vi "Read Digital Input and Output Module.vi"   [LabVIEW 2017, in "Scan Engine Scripting.lvlib"]
doc: "Returns the channel settings of a digital input and output module that can be edited and then used to create a new module instance to set into a slot."
uses:
  Scan Engine Scripting.lvlib
  NI 9375/NI 9375.lvclass
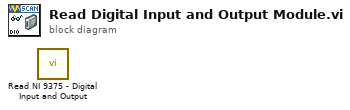
[diagram p0: block diagram]
diagram:
  n1 = call "Read NI 9375 - Digital Input and Output.vi"() -> ()  [unwired: 9 in, 3 out]
